vi "CreateSetupDUTDisplayData.vi"(7 "SMU":T2, 10 "SMU Data":dbl[][](array[numeric]), 11 "DUT Names":string[][](array[string])) -> (3 "DUT Display Data":T1[](array[typedef]) {"Resistance (Ohm)" format="%_4p"; "Current (A)" format="%_4p"; "Voltage (V)" format="%_4p"})   [LabVIEW 2012]
uses:
  driver/Public/Controls/SMU.ctl
  DUTDisplayData.ctl
  driver/Keithley-2602.lvlib
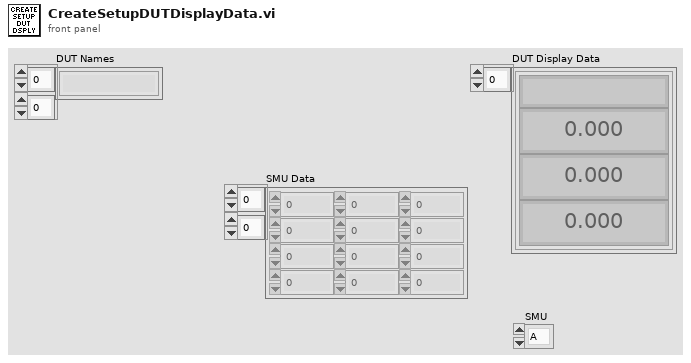
[diagram p1: front panel]
types:
  T1 = typedef "DUTDisplayData.ctl" = cluster{"Name":string, "Voltage (V)":dbl, "Current (A)":dbl, "Resistance (Ohm)":dbl}
  T2 = typedef "Keithley-2602.lvlib/SMU.ctl" = enum16{"A", "B"}
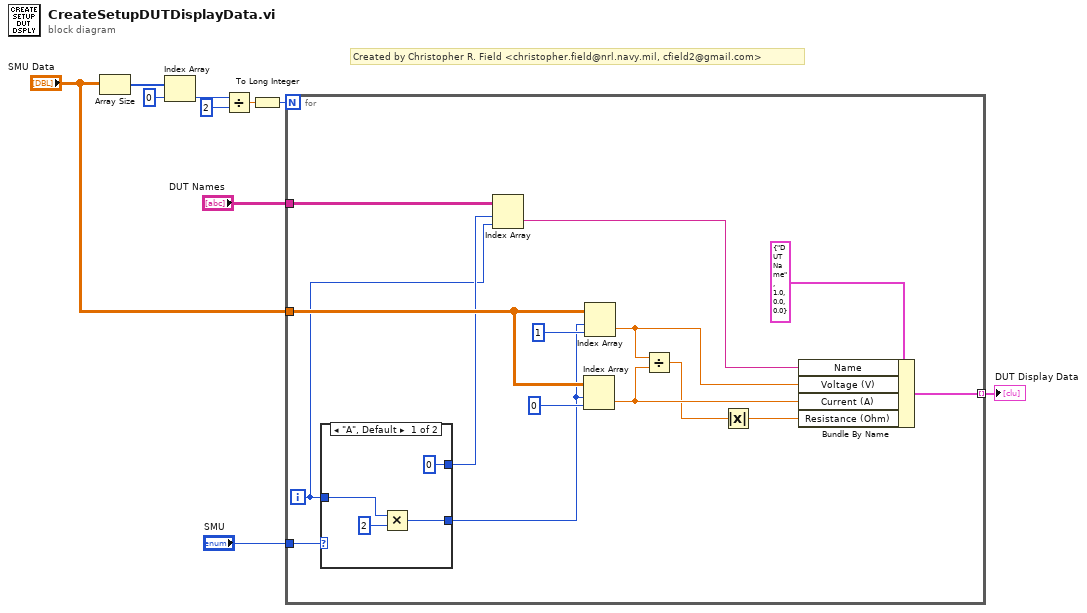
[diagram p0: block diagram]
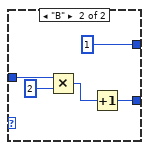
[diagram p2: hidden frame]
diagram:
  # "Created by Christopher R. Field <christopher.field@nrl.navy.mil, cfield2@gmail.com>"
  n1 = Array Size(array="SMU Data") -> (size(s)=w10:i32[])
  n2 = Index Array(array=w10, index=0) -> (element=w8:i32)
  n3 = Divide(x=w8, y=2) -> (x/y=w3:dbl)
  n4 = To Long Integer(number=w3) -> (32bit integer=w4:i32)
  n5 = for {
    N: w4 -> [_]
    tunnel: "SMU Data" -> [w25]
    tunnel: "SMU" -> [w22]
    tunnel: [w17] -> w1 mode=indexing
    tunnel: "DUT Names" -> [w16]
    i -> [w14]
    n6 = case shown="\"A\", Default" w22 {
      tunnel: [w28 w32] -> w21
      tunnel: w14 -> [w27 w34]
      tunnel: [0 1] -> w15
      frame "A", Default {
        n7 = Multiply(x=w27, y=u32 2) -> (x*y=w28:u32)
      }
      frame "B" {
        n8 = Multiply(x=w34, y=u32 2) -> (x*y=w31:u32)
        n9 = Increment(x=w31) -> (x+1=w32:u32)
      }
    }
    n10 = Index Array(array=w16, index (row)=w15, index (col)=w14) -> (element=w13:string)
    n11 = Index Array(array=w25, index (row)=w21, index (col)=0 ("disabled index (col)")) -> (element=w18:dbl)
    n12 = Index Array(array=w25, index (row)=w21, index (col)=1 ("disabled index (col)")) -> (element=w19:dbl)
    n13 = Divide(x=w19, y=w18) -> (x/y=w12:dbl)
    n14 = Absolute Value(x=w12) -> (abs(x)=w11:dbl)
    n15 = Bundle By Name(cluster=T1 {"Name"="DUT Name", "Voltage (V)"=1.0, "Current (A)"=0.0, "Resistance (Ohm)"=0.0} ("DUT Display Data"), "Name"=w13, "Voltage (V)"=w19, "Current (A)"=w18, "Resistance (Ohm)"=w11) -> (w17:T1)
  }
  "DUT Display Data" <- w1
